vi "01_DSP_zero_cross_detektor.vi"() -> ()   [LabVIEW 2019]
uses:
  <vilib>/Analysis/baseanly.llb/Mean (DBL).vi
  <vilib>/measure/NI_MABase.lvlib
  <vilib>/Analysis/NI_AALBase.lvlib
panel:
  out "Median frekvence (Hz)":dbl=9.709653092006032 format="%0.2f"
  out "Prumerna frekvence (Hz)":dbl=33.26345398264088 format="%0.2f"
  out "Frekvence signalu (Hz)":dbl[](array[numeric])=[9.80392156862745, 10.638297872340425, 4.9504950495049505, 9.615384615384617, 10.204081632653065, 5.050505050505049, 5.102040816326532, 124.99999999999989, 4.950495049504951, 5.102040816326526, 5.050505050505052, 9.803921568627464, 10.416666666666657, 249.99999999999977]
  out "Perioda signalu (s)":dbl[](array[numeric])=[0.10200000000000001, 0.094, 0.202, 0.10399999999999998, 0.09799999999999996, 0.19800000000000004, 0.19599999999999992, 0.008000000000000007, 0.20199999999999996, 0.19600000000000017, 0.19799999999999995, 0.10199999999999987, 0.09600000000000009, 0.0040000000000000036]
  out "Pole casu pruchodu nulou":dbl[](array[numeric])=[0.001, 0.052000000000000005, 0.099, 0.2, 0.252, 0.301, 0.4, 0.498, 0.502, 0.603, 0.7010000000000001, 0.8, 0.851, 0.899, 0.901]
  out "dt (s)":dbl=0.001
  out "Vzorkovaci Frekvence (N)":dbl=1000.0
  out "1_XY Graph":cluster{dbl[], dbl[]}[](graph)=[{array[1000 elements], array[1000 elements]}, {[0.001, 0.052000000000000005, 0.099, 0.2, 0.252, 0.301, 0.4, 0.498, 0.502, 0.603, 0.7010000000000001, 0.8, 0.851, 0.899, 0.901], [1.1413995323074777, 0.15555163258390536, 0.23003454822476, 0.5175309086225085, 0.06763131606118444, 1.2128297923760567, 0.16758325178737296, 0.08223938211899073, 1.0561810291308282, 1.6305843135033822, 0.07411340896042895, 0.6575699015767263, 0.5988568871389047, 0.2826793630094516, 0.8491341683128938]}]
  in  "Amplituda sumu":dbl=0.9999999999999999 format="%.2p"
  in  "Info o vzorkovani":T1={"Vzorkovaci frekvence"=1000.0, "Pocet vzorku v okne"=1000.0} {"Vzorkovaci frekvence" format="%.2p"}
  in  "Faze":dbl format="%.2p"
  in  "Amplituda":dbl=10.0 format="%0.2p"
  in  "Frekvence":dbl=10.0 format="%0.2p"
  # "GENEROVANI SIGNALU"
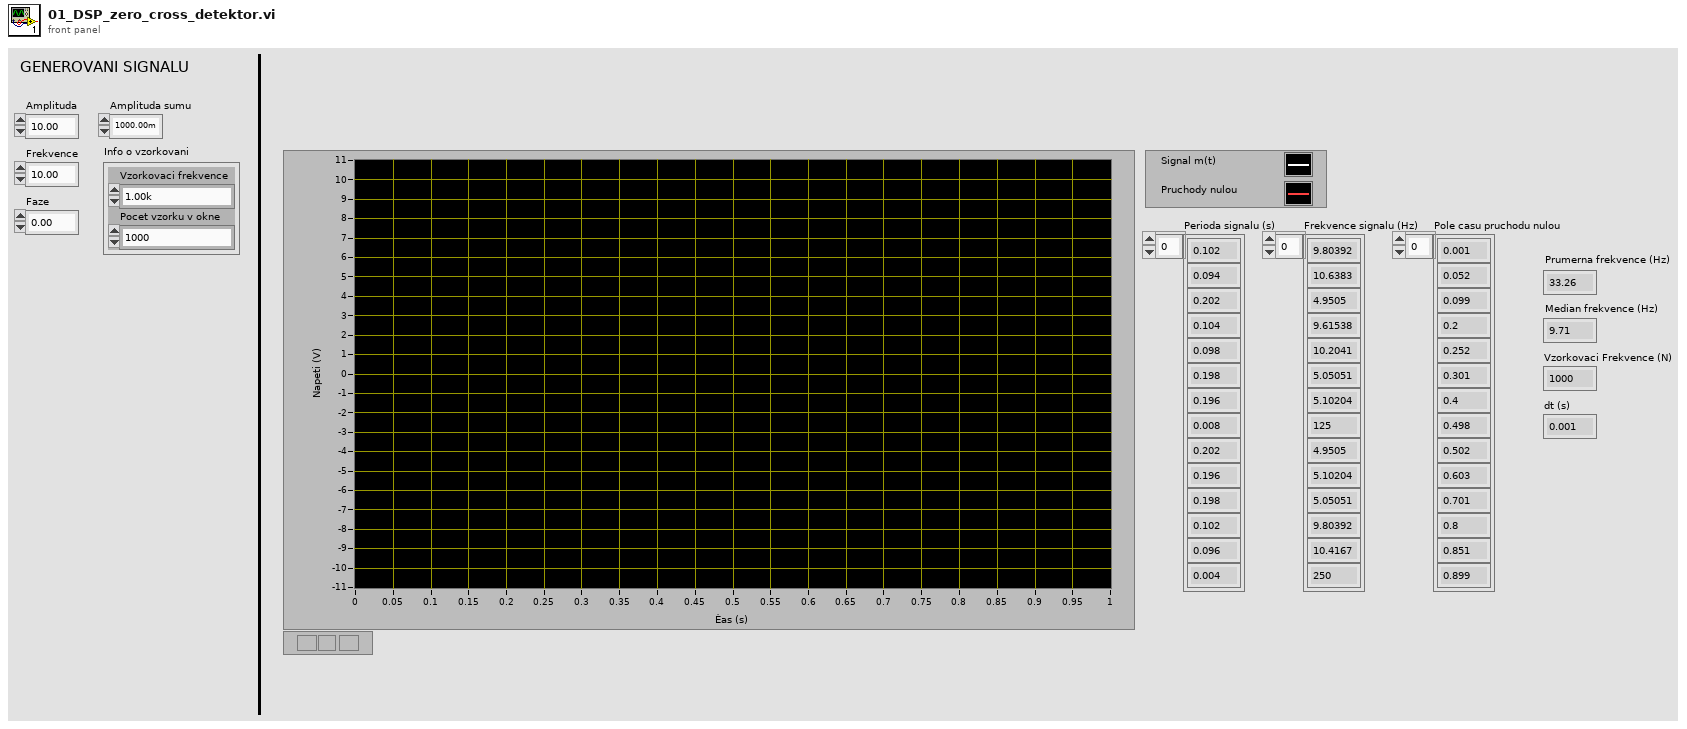
[diagram p1: front panel]
types:
  T1 = cluster{"Vzorkovaci frekvence":dbl, "Pocet vzorku v okne":dbl}
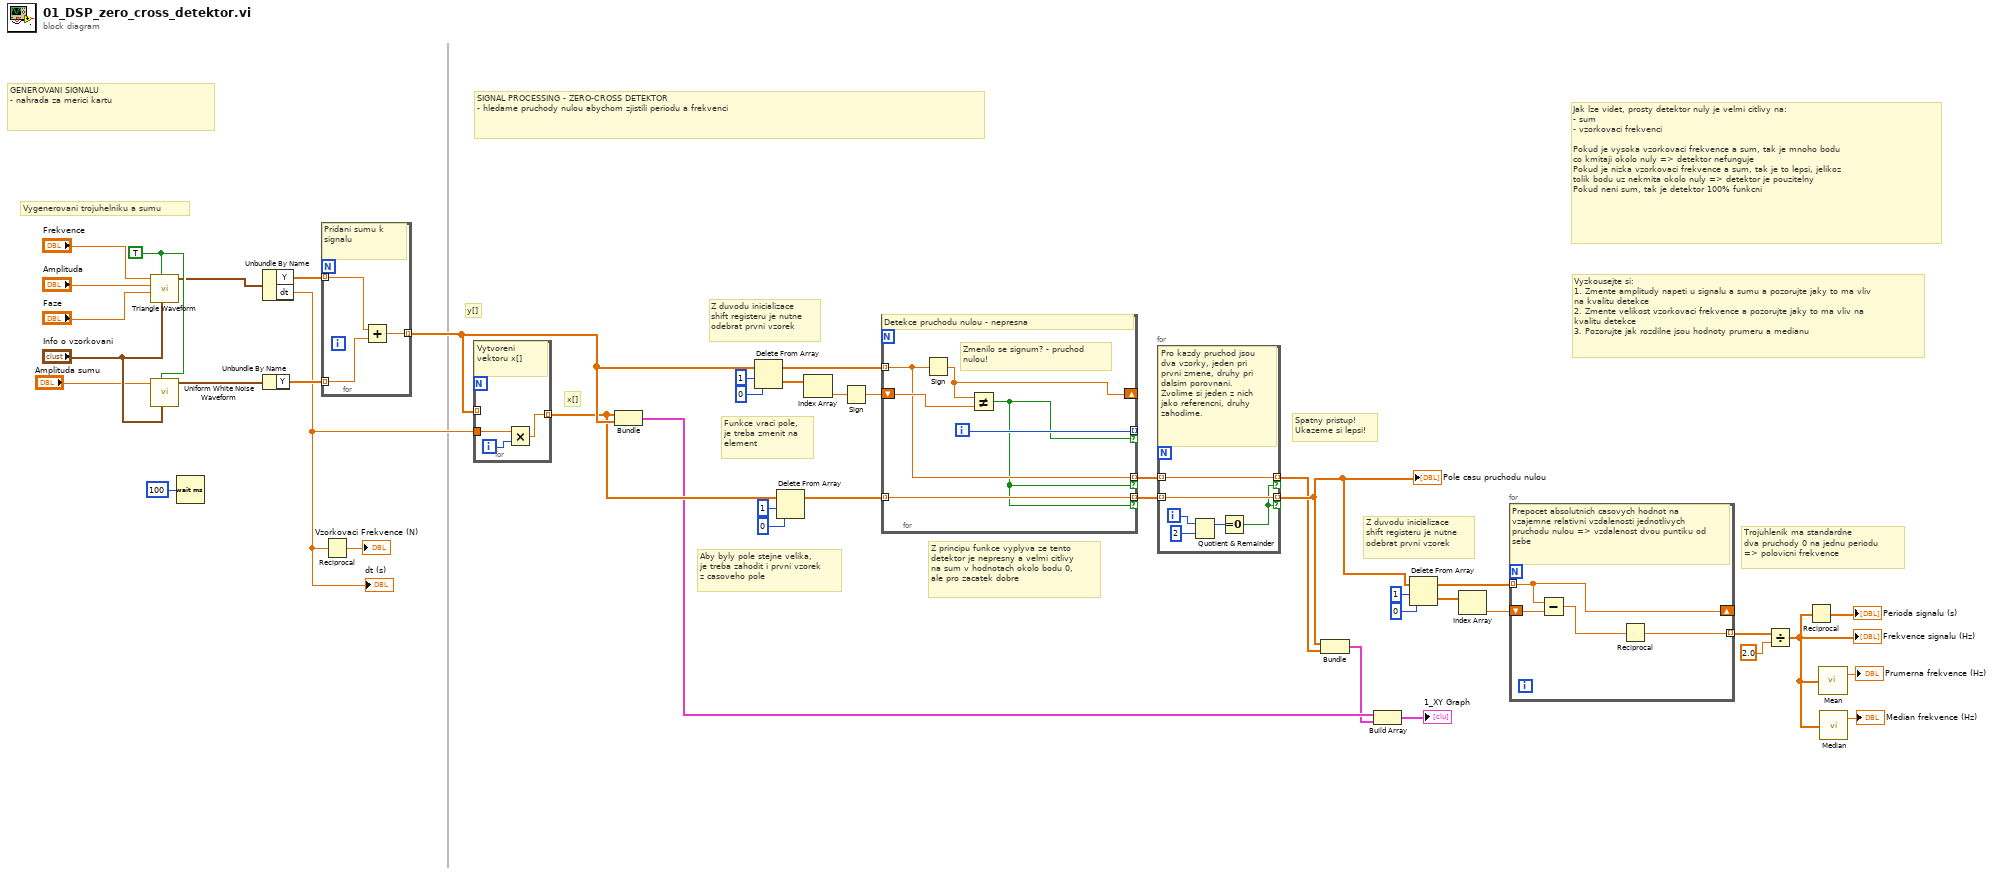
[diagram p0: block diagram]
diagram:
  w37 = TRUE ("reset signal")
  # "Spatny pristup!\nUkazeme si lepsi!"
  # "x[]"
  # "y[]"
  # "Vyzkousejte si:\n1. Zmente amplitudy napeti u signalu a sumu a pozorujte jaky to ma vliv \nna kvalitu detekce\n2. Zmente velikost vzorkovaci frekvence a pozorujte jaky to ma vliv na \nkvalitu detekce\n3. Pozorujte jak rozdilne jsou hodnoty prumeru a medianu"
  # "Jak lze videt, prosty detektor nuly je velmi citlivy na:\n- sum\n- vzorkovaci frekvenci\n\nPokud je vysoka vzorkovaci frekvence a sum, tak je mnoho bodu\nco kmitaji okolo nuly => detektor nefunguje\nPokud je nizka vzorkovaci frekvence a sum, tak je to lepsi, jelikoz\ntolik bodu uz nekmita okolo nuly => detektor je pouzitelny\nPokud neni sum, tak je detektor 100% funkcni"
  # "SIGNAL PROCESSING - ZERO-CROSS DETEKTOR\n- hledame pruchody nulou abychom zjistili periodu a frekvenci"
  # "GENEROVANI SIGNALU\n- nahrada za merici kartu"
  # "Trojuhlenik ma standardne \ndva pruchody 0 na jednu periodu\n=> polovicni frekvence"
  # "Z duvodu inicializace\nshift registeru je nutne\nodebrat prvni vzorek"
  # "Z principu funkce vyplyva ze tento\ndetektor je nepresny a velmi citlivy \nna sum v hodnotach okolo bodu 0,\nale pro zacatek dobre"
  # "Aby byly pole stejne velika,\nje treba zahodit i prvni vzorek\nz casoveho pole"
  # "Funkce vraci pole,\nje treba zmenit na \nelement"
  # "Z duvodu inicializace\nshift registeru je nutne\nodebrat prvni vzorek"
  # "Vygenerovani trojuhelniku a sumu"
  n1 = call <vilib>:"Triangle Waveform.vi"("sampling info"="Info o vzorkovani", "reset signal"=w37, "phase"="Faze", "amplitude"="Amplituda", "frequency"="Frekvence") -> ("signal out"=w33:waveform(dbl))  [unwired: 5 in, 1 out]
  n2 = call <vilib>:"Uniform White Noise Waveform.vi"("sampling info"="Info o vzorkovani", "reset signal"=w37, "amplitude"="Amplituda sumu") -> ("signal out"=w36:waveform(dbl))  [unwired: 7 in, 1 out]
  n3 = Wait (ms)(milliseconds to wait=u32 100) -> ()  [unwired: 1 out]
  n4 = Unbundle By Name(w33) -> ("Y"=w35:dbl[], "dt"=w32:dbl)
  "dt (s)" <- w32
  n5 = Unbundle By Name(w36) -> ("Y"=w34:dbl[])
  n6 = for {
    tunnel: w35 -> [w44] mode=indexing
    tunnel: w34 -> [w45] mode=indexing
    tunnel: [w43] -> w30 mode=indexing
    # "Pridani sumu k signalu"
    n7 = Add(x=w44, y=w45) -> (x+y=w43:dbl)
  }
  n8 = Reciprocal(x=w32) -> (1/x=→"Vzorkovaci Frekvence (N)":dbl)
  n9 = for {
    tunnel: w30 -> [_] mode=indexing
    tunnel: w32 -> [w47]
    tunnel: [w46] -> w22 mode=indexing
    i -> [w48]
    # "Vytvoreni vektoru x[]"
    n10 = Multiply(x=w47, y=w48) -> (x*y=w46:dbl)
  }
  n11 = Bundle(w22, w30) -> (w16:cluster{dbl[], dbl[]})  [unwired: 1 in]
  n12 = Delete From Array(array=w30, length=1, index=0) -> (deleted portion=w26:dbl[], array with subset deleted=w29:dbl[])
  n13 = Delete From Array(array=w22, length=1, index=0) -> (array with subset deleted=w23:dbl[])  [unwired: 1 out]
  n14 = Index Array(array=w26) -> (element=w9:dbl)  [unwired: 1 in]
  n15 = Sign(1:w9) -> (0:w8:dbl)
  n16 = for {
    tunnel: w29 -> [w50] mode=indexing
    shift-right: [w54] -> _
    shift-left: w8 -> [w53]
    tunnel: [w52] -> _ mode=indexing if=w49
    tunnel: w23 -> [w51] mode=indexing
    tunnel: [w51] -> w12 mode=indexing if=w49
    tunnel: [w50] -> w13 mode=indexing if=w49
    i -> [w52]
    # "Zmenilo se signum? - pruchod\nnulou!"
    # "Detekce pruchodu nulou - nepresna"
    n17 = Sign(1:w50) -> (0:w54:dbl)
    n18 = Not Equal?(x=w54, y=w53) -> (x != y?=w49:bool)
  }
  n19 = for {
    tunnel: w13 -> [w58] mode=indexing
    tunnel: w12 -> [w57] mode=indexing
    tunnel: [w58] -> w10 mode=indexing if=w55
    tunnel: [w57] -> w11 mode=indexing if=w55
    i -> [w60]
    # "Pro kazdy pruchod jsou dva vzorky, jeden pri prvni zmene, druhy pri dalsim porovnani.  Zvolime si jeden z nich jako referencni, druhy zahodime."
    n20 = Quotient & Remainder(x=w60, y=2) -> (x-y*floor(x/y)=w56:i32)  [unwired: 1 out]
    n21 = Equal To 0?(x=w56) -> (x = 0?=w55:bool)
  }
  "Pole casu pruchodu nulou" <- w11
  n22 = Bundle(w11, w10) -> (w15:cluster{dbl[], dbl[]})  [unwired: 1 in]
  n23 = Build Array(w16, w15) -> (→"1_XY Graph":cluster{dbl[], dbl[]}[])
  n24 = Delete From Array(array=w11, length=1, index=0) -> (deleted portion=w21:dbl[], array with subset deleted=w18:dbl[])
  n25 = Index Array(array=w21) -> (element=w17:dbl)  [unwired: 1 in]
  n26 = for {
    tunnel: w18 -> [w64] mode=indexing
    shift-right: [w64] -> _
    shift-left: w17 -> [w63]
    tunnel: [w61] -> w7 mode=indexing
    # "Prepocet absolutnich casovych hodnot na vzajemne relativni vzdalenosti jednotlivych pruchodu nulou => vzdalenost dvou puntiku od sebe"
    n27 = Subtract(x=w64, y=w63) -> (x-y=w62:dbl)
    n28 = Reciprocal(x=w62) -> (1/x=w61:dbl)
  }
  n29 = Divide(x=w7, y=2.0) -> (x/y=w4:dbl[])
  "Frekvence signalu (Hz)" <- w4
  n30 = Reciprocal(x=w4) -> (1/x=→"Perioda signalu (s)":dbl[])
  n31 = call-poly <vilib>:"Mean.vi"("X"=w4) -> ("mean"=→"Prumerna frekvence (Hz)":dbl)  [unwired: 1 out]
  n32 = call <vilib>:"Median.vi"("X"=w4) -> ("median"=→"Median frekvence (Hz)":dbl)  [unwired: 1 out]
